vi "NeedRecalcPath.vi"(0 "Project":T1, 4 "ignoreBall?":bool, 5 "Initial State":dbl[](array[numeric]), 6 "SmoothPath":dbl[][](array[numeric]), 7 "Pos x,y":dbl[](array[numeric]), 8 "Volta ao redor\nda área?":bool, 9 "IA State":T2={"our_robots"=[], "enemy_robots"=[], "balls"=[], "geometry"={"line_width"=0, "field_length"=0, "field_width"=0, "boundary_width"=0, "referee_width"=0, "goal_width"=0, "goal_depth"=0, "goal_wall_width"=0, "center_circle_radius"=0, "defense_radius"=0, "defense_stretch"=0, "free_kick_from_defense_dist"=0, "penalty_spot_from_field_line_dist"=0, "penalty_line_from_spot_dist"=0}, "IA Judge"={"stage"="", "command"="", "our_goalie_id"=0.0, "enemy_goalie_id"=0.0, "command enum"=enum."Halt", "Time"=enum."Azul"}, "Received Timestamp"=timestamp(0 s since 1904-01-01), "Events"={"Touch"=FALSE, "Ball out"=FALSE, "id touch"=0.0, "Ball out of \nVision"=FALSE, "Ball inside \nGoalie area"=FALSE, "Robot not responding"=FALSE, "Robots responding status"=[1.0, 1.0, 1.0, 1.0, 1.0, 1.0], "Enemy Ball \nPossession"=FALSE, "Pass State"=FALSE, "id end of pass"=0.0, "Kick"=FALSE, "Id ini Possession"=0.0, "Ball Possesion"=FALSE, "Id Possesion"=0.0, "Direct Kick"=FALSE, "2nd Strk Ativo"=FALSE}}, 10 "Robot":T3={"id"=0, "function"=enum."Attacker", "x"=0.0, "y"=0.0, "orientation"=0.0, "v_tangent"=0.0, "v_normal"=0.0, "v_ang"=0.0, "kick_x"=0.0, "kick_z"=0.0, "dribble"=FALSE, "Timestamp"=timestamp(0 s since 1904-01-01), "estimatives"={"est_v_tangent"=0.0, "est_v_normal"=0.0, "est_vx"=0.0, "est_vy"=0.0, "Pos Robot Est"=[]}, "dest_x_kick"=0.0, "dest_y_kick"=0.0, "Gap Coord"=[], "States"=enum."Pass", "Path "=[], "Path  Smooth"=[], "Dest"=[], "vx_desired"=0.0, "vy_desired"=0.0, "slowBehavior"=FALSE, "VSSStates"=enum."Pass"}, 11 "Dest x,y":dbl[](array[numeric])) -> (2 "result":bool, 3 "NeedRecalc":bool)   [LabVIEW 2023]
uses:
  Vision_class/Old vision/Controls/AI Robot.ctl
  Vision_class/Old vision/Controls/Functions Enum.ctl
  Vision_class/Old vision/Controls/AttackerStates.ctl
  Vision_class/Old vision/Controls/PathDests.ctl
  Vision_class/Old vision/Controls/PathDest.ctl
  Navigation/VSSNavigation/VSSAttackerStates.ctl
  Vision_class/Old vision/SSL Detection Frame Simple Estimator Cameras VelCmd Folder/Core/AI Input.ctl
  Vision_class/Old vision/SSL Detection Frame Simple Estimator Cameras VelCmd Folder/Core/AI Ball.ctl
  Vision_class/Old vision/SSL Detection Frame Simple Estimator Cameras VelCmd Folder/Core/Field Size.ctl
  Vision_class/Old vision/SSL Detection Frame Simple Estimator Cameras VelCmd Folder/Core/AI Judge.ctl
  Communication_class/Paths/MessageAI_State Folder/Intel/Command Enum.ctl
  Vision_class/Old vision/SSL Detection Frame Simple Estimator Cameras VelCmd Folder/Util/Events/Events.ctl
  Parameters_class/Project.ctl
  <vilib>/Analysis/_algsub.llb/Real Vector Norm.vi
  <vilib>/Analysis/NI_AALPro.lvlib
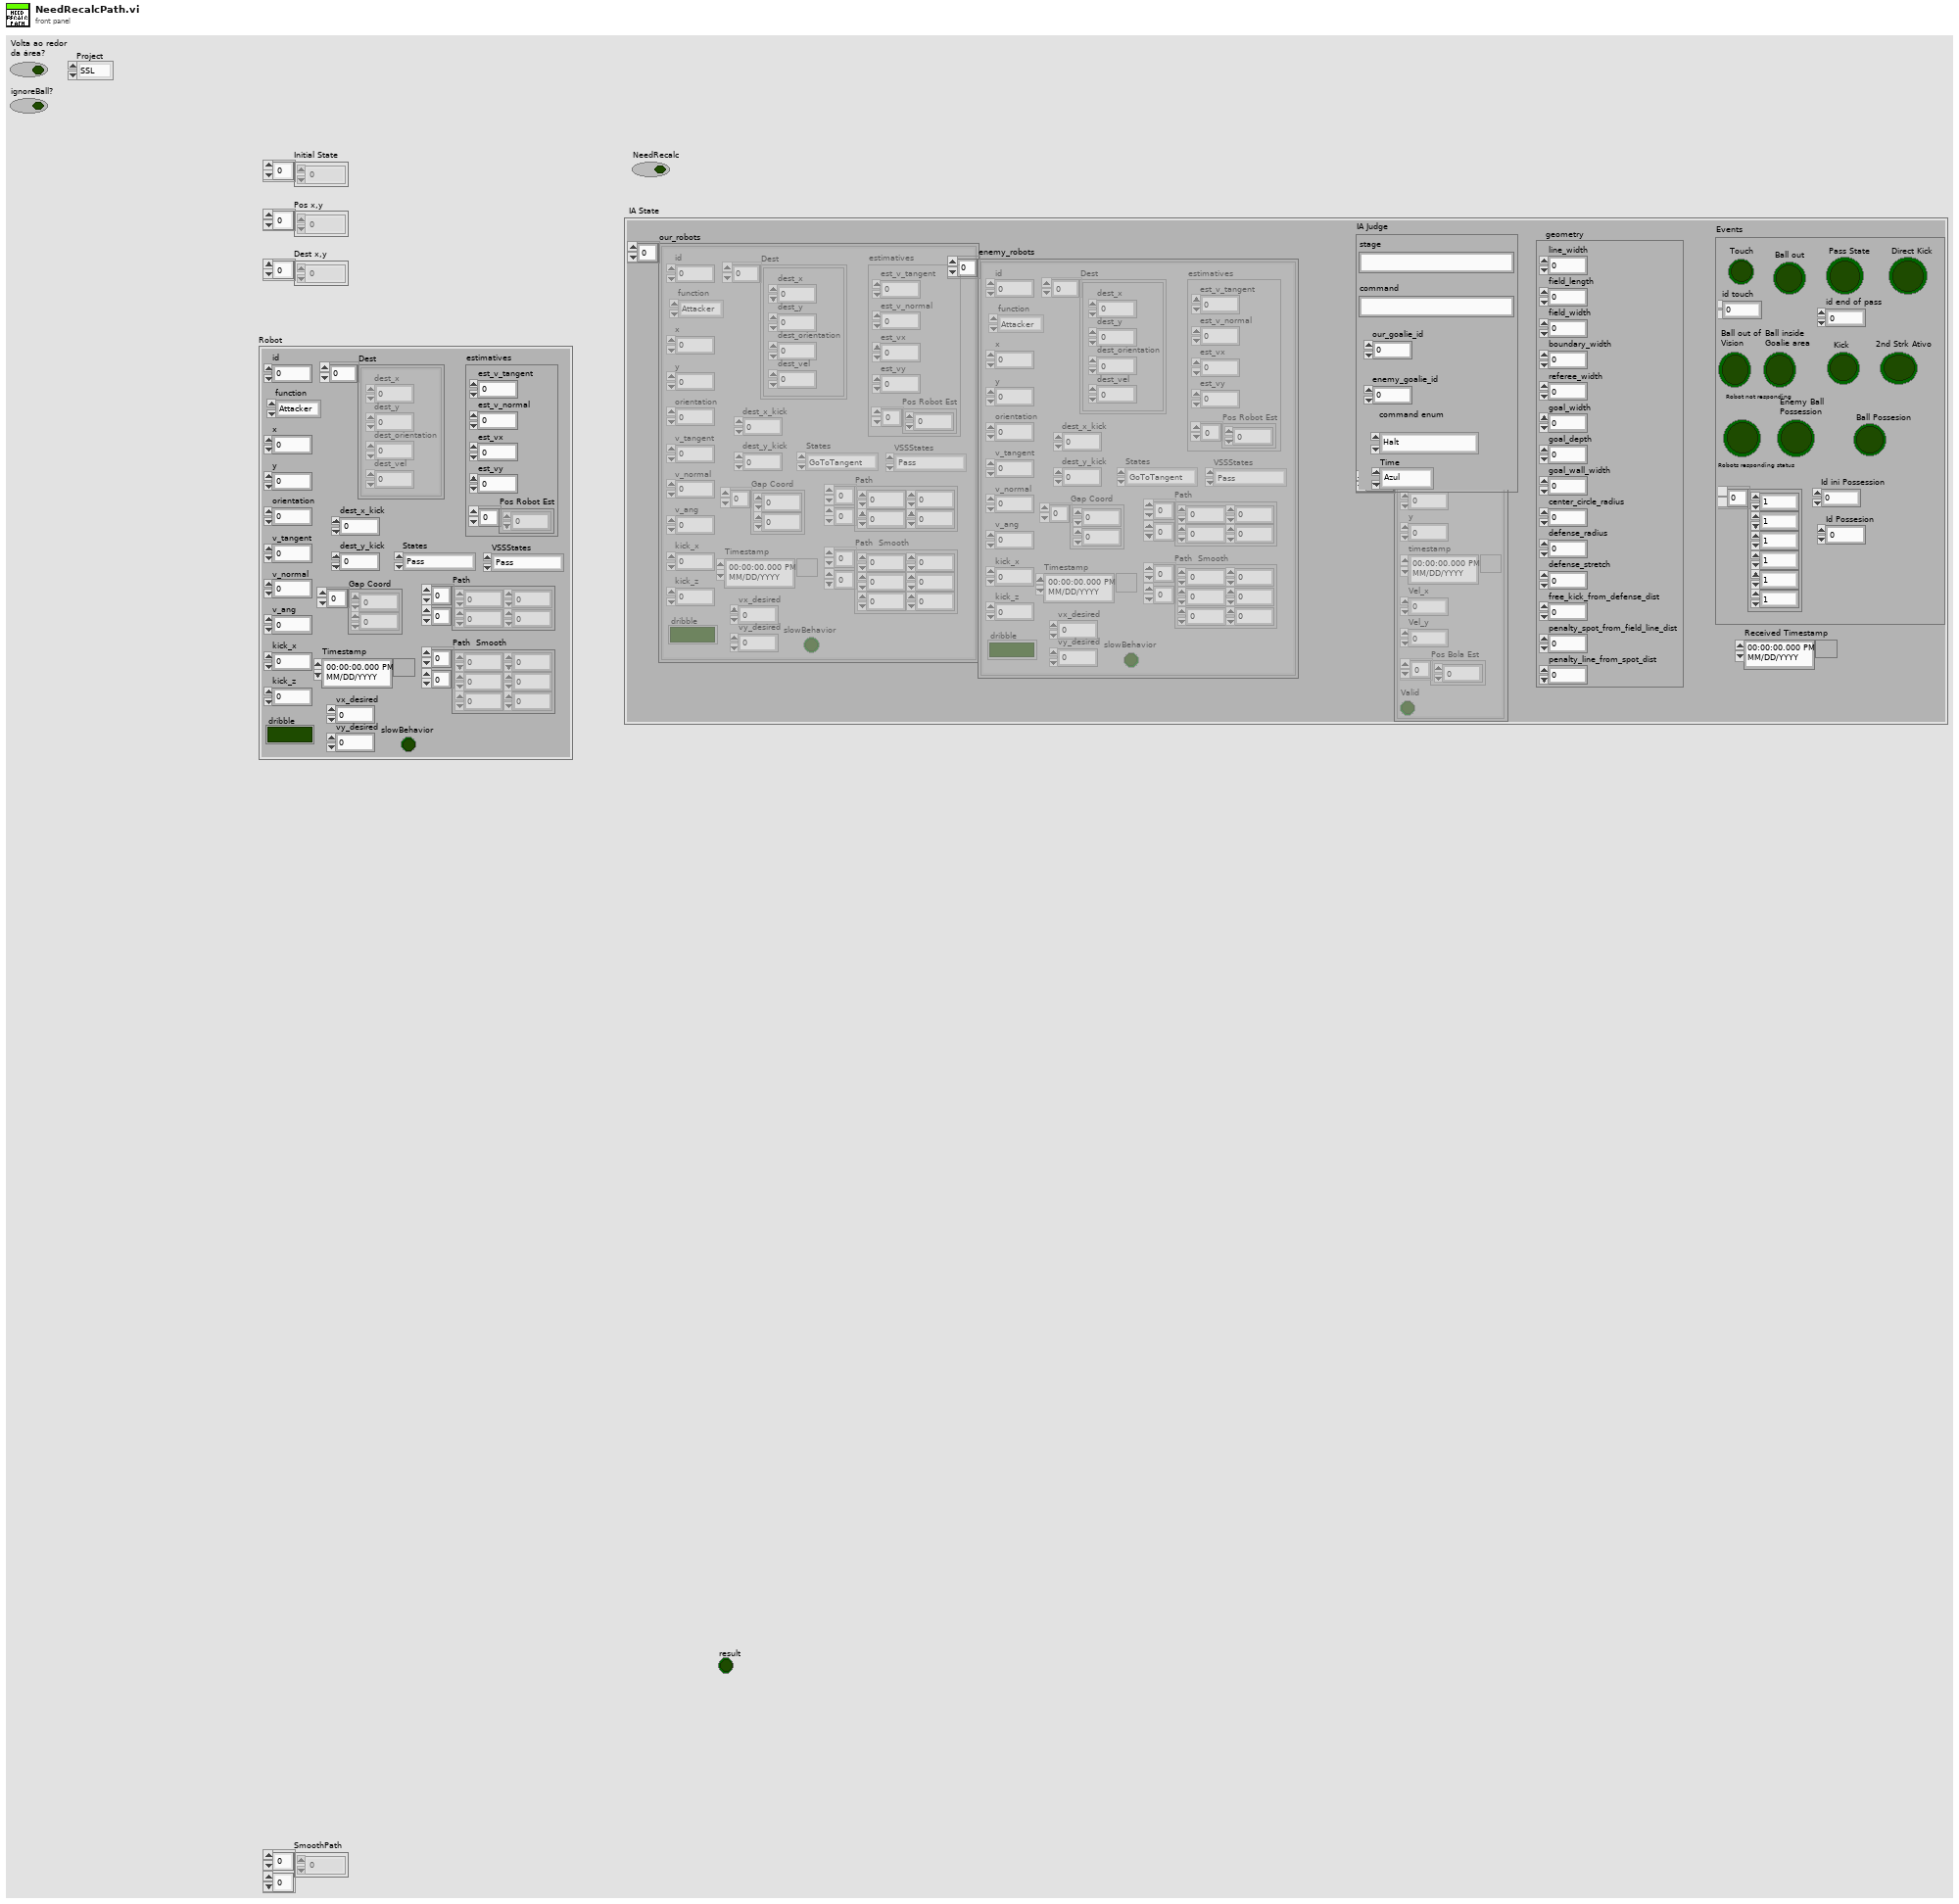
[diagram p1: front panel]
types:
  T1 = typedef "Project.ctl" = enum16{"SSL", "VSS"}
  T2 = typedef "AI Input.ctl" = cluster{"our_robots":T3[], "enemy_robots":T3[], "balls":T9[], "geometry":T10, "IA Judge":T11, "Received Timestamp":timestamp, "Events":T13}
  T3 = typedef "AI Robot.ctl" = cluster{"id":u32, "function":T4, "x":dbl, "y":dbl, "orientation":dbl, "v_tangent":dbl, "v_normal":dbl, "v_ang":dbl, "kick_x":dbl, "kick_z":dbl, "dribble":bool, "Timestamp":timestamp, "estimatives":cluster{"est_v_tangent":dbl, "est_v_normal":dbl, "est_vx":dbl, "est_vy":dbl, "Pos Robot Est":dbl[]}, "dest_x_kick":dbl, "dest_y_kick":dbl, "Gap Coord":dbl[], "States":T5, "Path ":dbl[][], "Path  Smooth":dbl[][], "Dest":T6, "vx_desired":dbl, "vy_desired":dbl, "slowBehavior":bool, "VSSStates":T8}
  T4 = typedef "Functions Enum.ctl" = enum16{"2nd Striker", "Attacker", "Goalie", "Defender", "Striker", "Goto 0", "Dummy", "Kicker", "ZigZag 0", "ZigZag 1", "ZigZag 2", "ZigZag 3", "ZigZag 4", "ZigZag 5", "ZigZag 6", "ZigZag 7", "ZigZag 8", ""}
  T5 = typedef "AttackerStates.ctl" = enum16{"Pass", "GoToTangent", "BallGetting", "GoToKick", ""}
  T6 = typedef "PathDests.ctl" = T7[]
  T7 = typedef "PathDest.ctl" = cluster{"dest_x":dbl, "dest_y":dbl, "dest_orientation":dbl, "dest_vel":dbl}
  T8 = typedef "VSSAttackerStates.ctl" = enum16{"Pass", "GoToTangent", "BallGetting", "GoToKick", "Rotate anti-clockwise", "Rotate Clockwise", ""}
  T9 = typedef "AI Ball.ctl" = cluster{"x":dbl, "y":dbl, "timestamp":timestamp, "Vel_x":dbl, "Vel_y":dbl, "Pos Bola Est":dbl[], "Valid":bool}
  T10 = typedef "Field Size.ctl" = cluster{"line_width":u32, "field_length":u32, "field_width":u32, "boundary_width":u32, "referee_width":u32, "goal_width":u32, "goal_depth":u32, "goal_wall_width":u32, "center_circle_radius":u32, "defense_radius":u32, "defense_stretch":u32, "free_kick_from_defense_dist":u32, "penalty_spot_from_field_line_dist":u32, "penalty_line_from_spot_dist":u32}
  T11 = typedef "AI Judge.ctl" = cluster{"stage":string, "command":string, "our_goalie_id":dbl, "enemy_goalie_id":dbl, "command enum":T12, "Time":enum16{"Azul", "Amarelo"}}
  T12 = typedef "Command Enum.ctl" = enum16{"Halt", "Stop", "Force Start", "PKA Normal Start", "Prepare Kickoff Ally", "PKE Normal Start", "Prepare Kickoff Enemy", "Prepare Penalty Ally", "PPA Normal Start", "Prepare Penalty Enemy", "PPE Normal Start", "Direct Free Enemy", "Direct Free Ally", "Indirect Free Enemy", "Indirect Free Ally", "Timeout Enemy", "Timeout Ally", "Goal Enemy", "Goal Ally", "Ball Placement Enemy", "Ball Placement Ally", "Normal Half Time", "Extra Time Break", "Extra Half Time", "None", "Post Game"}
  T13 = typedef "Events.ctl" = cluster{"Touch":bool, "Ball out":bool, "id touch":dbl, "Ball out of \nVision":bool, "Ball inside \nGoalie area":bool, "Robot not responding":bool, "Robots responding status":dbl[], "Enemy Ball \nPossession":bool, "Pass State":bool, "id end of pass":dbl, "Kick":bool, "Id ini Possession":dbl, "Ball Possesion":bool, "Id Possesion":dbl, "Direct Kick":bool, "2nd Strk Ativo":bool}
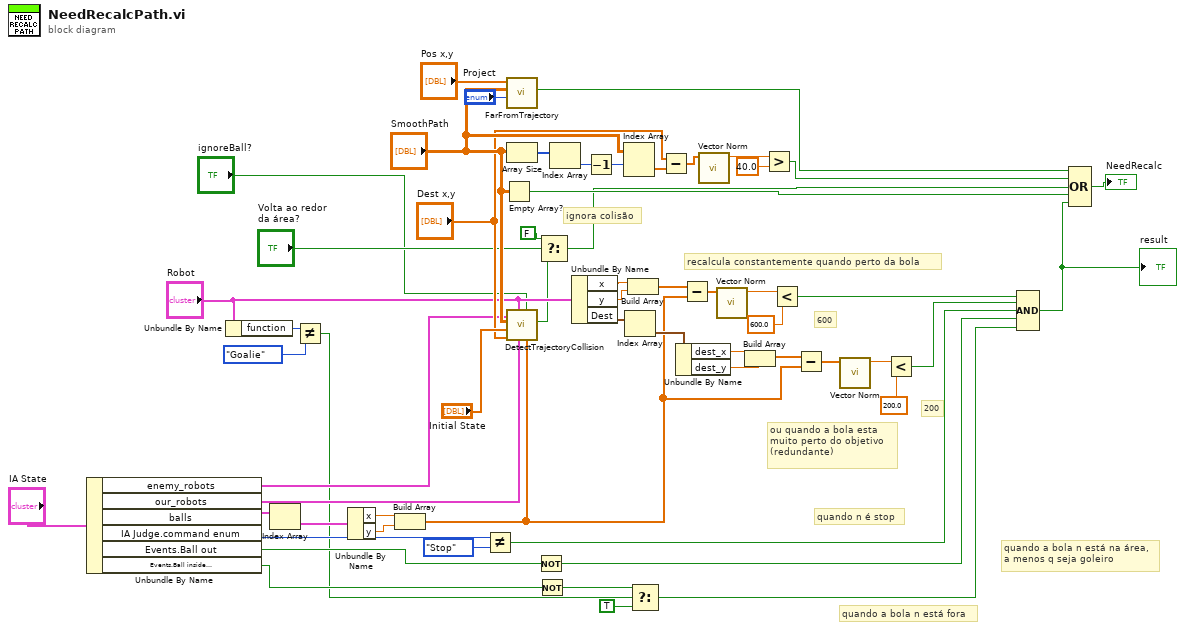
[diagram p0: block diagram]
diagram:
  # "ignora colisão"
  # "200"
  # "600"
  # "ou quando a bola esta\nmuito perto do objetivo\n(redundante)"
  # "quando a bola n está na área,\na menos q seja goleiro"
  # "quando n é stop"
  # "quando a bola n está fora"
  # "recalcula constantemente quando perto da bola"
  n1 = Unbundle By Name("IA State") -> ("enemy_robots"=w43:T3[], "our_robots"=w42:T3[], "balls"=w41:T9[], "IA Judge.command enum"=w22:T12, "Events.Ball out"=w17:bool, "Events.Ball inside \nGoalie area"=w12:bool)
  n2 = Unbundle By Name("Robot") -> ("function"=w19:T4)
  n3 = Index Array(array=w41) -> (element=w40:T9)  [unwired: 1 in]
  n4 = Not Equal?(x=w19, y=Functions_Enum."Goalie") -> (x != y?=w10:bool)
  n5 = Unbundle By Name(w40) -> ("x"=w36:dbl, "y"=w35:dbl)
  n6 = Build Array(w36, w35) -> (w23:dbl[])
  n7 = Not Equal?(x=w22, y=Command_Enum."Stop") -> (x != y?=w14:bool)
  n8 = Empty Array?(array="SmoothPath") -> (empty?=w54:bool)
  n9 = call "FarFromTrajectory.vi"("Project"="Project", "Path"="SmoothPath", "Position"="Pos x,y") -> ("Far from trajectory?"=w56:bool)  [unwired: 8 in]
  n10 = Array Size(array="SmoothPath") -> (size(s)=w45:i32[])
  n11 = call "DetectTrajectoryCollision.vi"("ball"=w23, "ignoreBall?"="ignoreBall?", "our_robots"=w42, "Robot in"="Robot", "Goal"="Dest x,y", "Initial State"="Initial State", "Last Path"="SmoothPath", "enemy_robots"=w43) -> ("Collision"=w5:bool)  [unwired: 3 in]
  n12 = Not(x=w17) -> (.not. x?=w13:bool)
  n13 = Not(x=w12) -> (.not. x?=w11:bool)
  n14 = Select(t=FALSE, s="Volta ao redor\nda área?", f=w5) -> (s? t:f=w4:bool)
  n15 = Index Array(array=w45) -> (element=w52:i32)  [unwired: 1 in]
  n16 = Unbundle By Name("Robot") -> ("x"=w39:dbl, "y"=w38:dbl, "Dest"=w32:T6)
  n17 = Decrement(x=w52) -> (x-1=w51:i32)
  n18 = Index Array(array="SmoothPath", index (row)=w51) -> (element=w46:dbl[])  [unwired: 1 in]
  n19 = Index Array(array=w32) -> (element=w31:T7)  [unwired: 1 in]
  n20 = Build Array(w39, w38) -> (w37:dbl[])
  n21 = Select(t=w11, s=w10, f=TRUE) -> (s? t:f=w8:bool)
  n22 = Subtract(x="Dest x,y", y=w46) -> (x-y=w47:dbl[])
  n23 = Unbundle By Name(w31) -> ("dest_x"=w29:dbl, "dest_y"=w28:dbl)
  n24 = Subtract(x=w37, y=w23) -> (x-y=w34:dbl[])
  n25 = call-poly <vilib>:"Vector Norm.vi"("Input Vector"=w47) -> ("norm"=w48:dbl)  [unwired: 9 in, 1 out]
  n26 = call-poly <vilib>:"Vector Norm.vi"("Input Vector"=w34) -> ("norm"=w33:dbl)  [unwired: 9 in, 1 out]
  n27 = Build Array(w29, w28) -> (w24:dbl[])
  n28 = Greater?(x=w48, y=40.0) -> (0:w49:bool)
  n29 = Less?(x=w33, y=600.0) -> (x < y?=w7:bool)
  n30 = Subtract(x=w24, y=w23) -> (x-y=w25:dbl[])
  n31 = call-poly <vilib>:"Vector Norm.vi"("Input Vector"=w25) -> ("norm"=w26:dbl)  [unwired: 9 in, 1 out]
  n32 = Less?(x=w26, y=200.0) -> (x < y?=w15:bool)
  n33 = Compound Arithmetic op=AND(w7, w15, w14, w13, w8) -> (w16:bool)
  "result" <- w16
  n34 = Compound Arithmetic op=OR(w56, w49, w4, w54, w16) -> (→"NeedRecalc":bool)
